vi "PUT.vi"(6 "timeout":i32=10000, 7 "output file":path, 8 "error in":errorcluster, 9 "buffer":string, 10 "url":string, 11 "http-client in":refnum<class "http-client.lvclass">) -> (0 "error out":errorcluster, 1 "body":string, 2 "headers":string, 3 "http-client out":refnum<class "http-client.lvclass">, 4 "status code":u16)   [LabVIEW 2025, in "http-client.lvclass"]
uses:
  http-client.lvclass
  REST Client/REST Client.lvclass
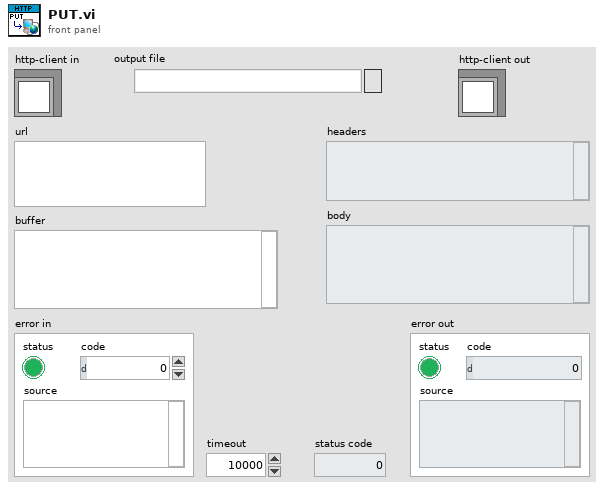
[diagram p1: front panel]
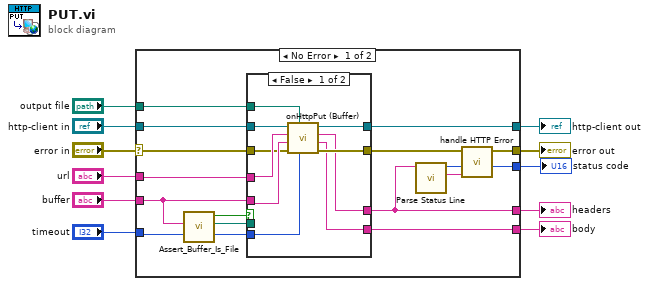
[diagram p0: block diagram]
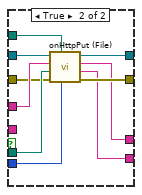
[diagram p2: hidden frame]
diagram:
  n1 = case shown="No Error" "error in" {
    selector: "error in" -> [w18 w49]
    tunnel: [w15 w49] -> w10
    tunnel: [w22 w48] -> w8
    tunnel: "http-client in" -> [w24 w48]
    tunnel: [w17 _] -> w7
    tunnel: "url" -> [w19 _]
    tunnel: "timeout" -> [w20 _]
    tunnel: "output file" -> [w23 _]
    tunnel: [w21 _] -> w3
    tunnel: "buffer" -> [w25 _]
    tunnel: [w13 _] -> w1
    frame No Error {
      n2 = call "Assert_Buffer_Is_File.vi"("body"=w25) -> ("File"=w26:path, "is File?"=w27:bool)  [unwired: 9 in]
      n3 = case shown="False" w27 {
        tunnel: w26 -> [_ w44]
        tunnel: w25 -> [w30 _]
        tunnel: w24 -> [w28 w46]
        tunnel: w23 -> [w36 w47]
        tunnel: [w37 w38] -> w22
        tunnel: [w32 w39] -> w17
        tunnel: [w33 w40] -> w21
        tunnel: w20 -> [w35 w43]
        tunnel: w19 -> [w31 w45]
        tunnel: [w34 w41] -> w16
        tunnel: w18 -> [w29 w42]
        frame False {
          n4 = call-dynamic "onHttpPut (Buffer).vi"("timeout"=w35, "output file"=w36, "error in"=w29, "buffer"=w30, "url"=w31, "http-method in"=w28) -> ("error out"=w34:errorcluster, "body"=w33:string, "headers"=w32:string, "http-method out"=w37:refnum<class "http-client.lvclass">)  [unwired: 2 in]
        }
        frame True {
          n5 = call-dynamic "onHttpPut (File).vi"("timeout"=w43, "output file"=w47, "error in"=w42, "file"=w44, "url"=w45, "http-method in"=w46) -> ("error out"=w41:errorcluster, "body"=w40:string, "headers"=w39:string, "http-method out"=w38:refnum<class "http-client.lvclass">)  [unwired: 2 in]
        }
      }
      n6 = call "Parse Status Line.vi"("Headers w/ status line"=w17) -> ("Status String"=w12:string, "status code"=w14:u16)  [unwired: 6 in, 3 out]
      n7 = call "handle HTTP Error.vi"("Status String"=w12, "status code"=w14, "error in (no error)"=w16) -> ("status code dup"=w13:u16, "error out"=w15:errorcluster)  [unwired: 7 in]
    }
    frame Error {
    }
  }
  "error out" <- w10
  "http-client out" <- w8
  "headers" <- w7
  "body" <- w3
  "status code" <- w1
